vi "_add value.vi"(6 "label":T1, 8 "i":errorcluster, 10 "B":refnum<class "Value.lvclass">, 11 "A":refnum<class "Value.lvclass">) -> (0 "error out":errorcluster, 2 "c":refnum<class "Value.lvclass">, 3 "A out":refnum<class "Value.lvclass">)   [LabVIEW 2023, in "LabGRAD.lvlib" / "Value.lvclass"]
uses:
  Value.lvclass
  UiObjects/string control.ctl
  operation.ctl
  Value.lvclass/Value.ctl
  UiObjects/UiObjects.lvclass
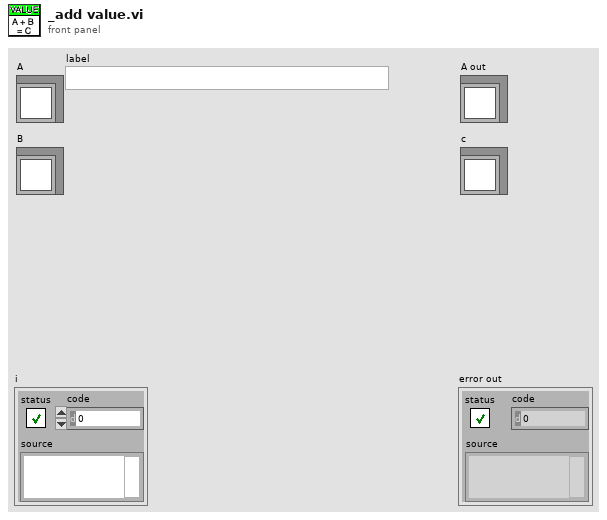
[diagram p1: front panel]
types:
  T1 = typedef "UiObjects.lvlib/UiObjects.lvclass/string control.ctl" = string
  T2 = typedef "LabGRAD.lvlib/Value.lvclass/operation.ctl" = enum16{"nop", "add", "subtract", "power", "multiply", "divide", "tanh"}
  T3 = typedef "UiObjects.lvlib/UiObjects.lvclass/numeric value control.ctl" = dbl
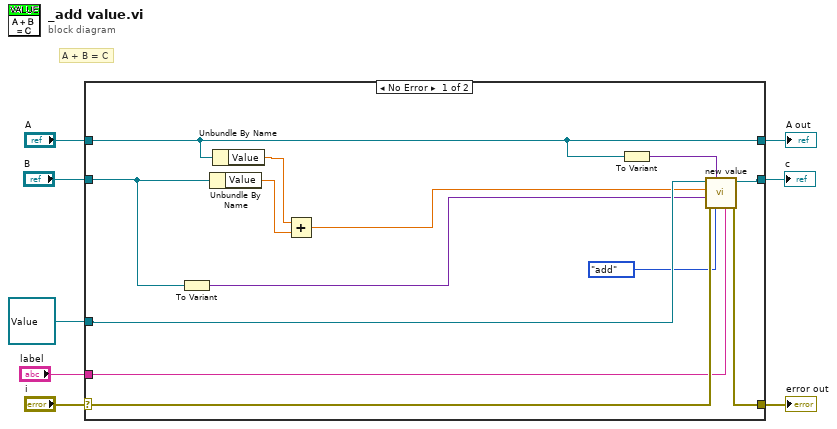
[diagram p0: block diagram]
diagram:
  # "A + B = C"
  n1 = case shown="No Error" "i" {
    selector: "i" -> [w12 w24]
    tunnel: [w11 w24] -> w7
    tunnel: [w15 w23] -> w5
    tunnel: "A" -> [w15 w23]
    tunnel: "B" -> [w19 _]
    tunnel: [w13 w22] -> w3
    tunnel: refnum<class "Value.lvclass"> refnum ("B") -> [w18 w22]
    tunnel: "label" -> [w9 _]
    frame No Error {
      n2 = To Variant(anything=w19) -> (Variant=w16:variant)
      n3 = Unbundle By Name(w19) -> ("Value"=w20:T3)
      n4 = Unbundle By Name(w15) -> ("Value"=w21:T3)
      n5 = Add(x=w21, y=w20) -> (x+y=w17:T3)
      n6 = To Variant(anything=w15) -> (Variant=w14:variant)
      n7 = call "new value.vi"("Label"=w9, "operation"=operation."add", "Previous"=w14, "error in (no error)"=w12, "Other"=w16, "data"=w17, "Value in"=w18) -> ("error out"=w11:errorcluster, "Value out"=w13:refnum<class "Value.lvclass">)  [unwired: 3 in]
    }
    frame Error {
    }
  }
  "error out" <- w7
  "A out" <- w5
  "c" <- w3
